vi "Set Admin Password.vi"(8 "error in (no error)":errorcluster, 10 "Set New Admin Password":T1, 11 "Master in":refnum<class "Master.lvclass">) -> (0 "error out":errorcluster, 3 "Master out":refnum<class "Master.lvclass">)   [LabVIEW 2014, in "Master.lvclass"]
uses:
  Master/Master.lvclass
  Master/Master.lvclass/Master.ctl
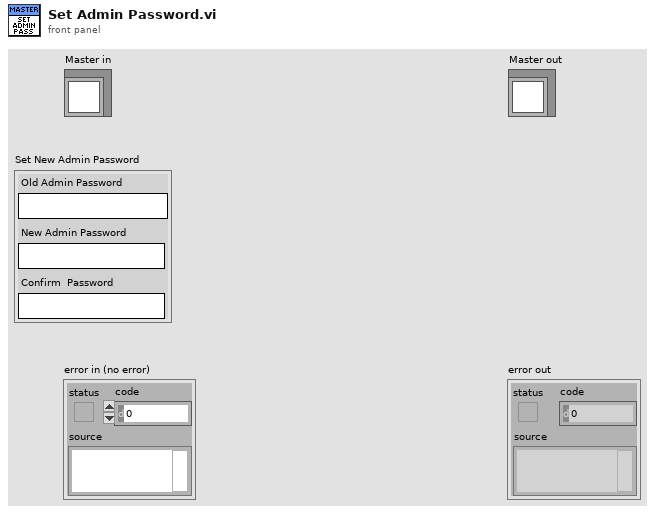
[diagram p1: front panel]
types:
  T1 = cluster{"Old Admin Password":string, "New Admin Password":string, "Confirm  Password":string}
  T2 = cluster{"Admin Password":string, "AutoLogoff":dbl}
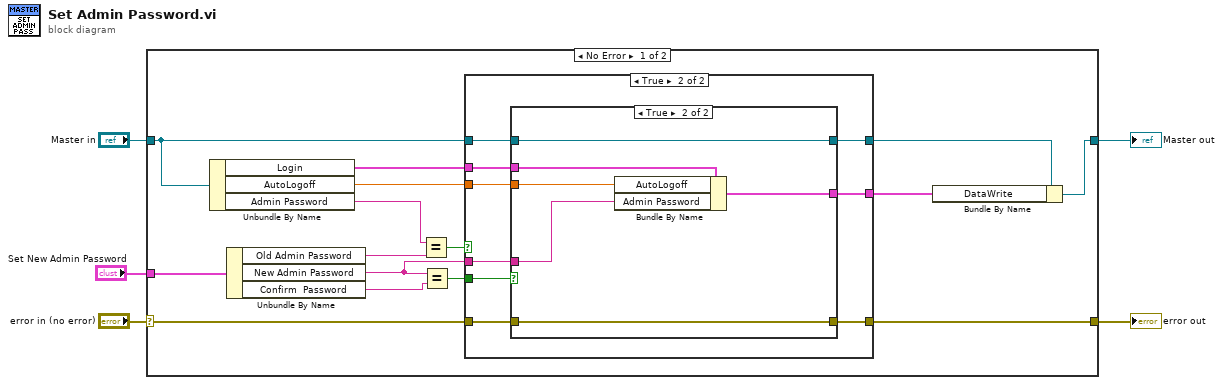
[diagram p0: block diagram]
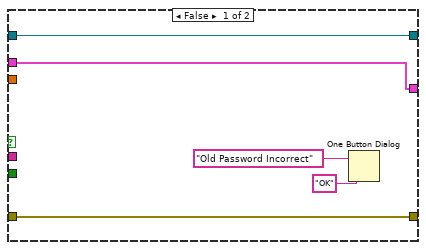
[diagram p2: hidden frame]
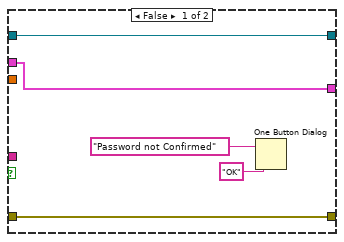
[diagram p3: hidden frame]
diagram:
  n1 = case shown="No Error" "error in (no error)" {
    selector: "error in (no error)" -> [w20 w47]
    tunnel: [w19 w47] -> w4
    tunnel: [w10 w46] -> w2
    tunnel: "Master in" -> [w17 w46]
    tunnel: "Set New Admin Password" -> [w18 _]
    frame No Error {
      n2 = Unbundle By Name(w17) -> ("Login"=w9:T2, "AutoLogoff"=w6:dbl, "Admin Password"=w7:string)
      n3 = Unbundle By Name(w18) -> ("Old Admin Password"=w16:string, "New Admin Password"=w12:string, "Confirm  Password"=w14:string)
      n4 = Equal?(x=w7, y=w16) -> (x = y?=w15:bool)
      n5 = Equal?(x=w12, y=w14) -> (x = y?=w13:bool)
      n6 = case shown="True" w15 {
        tunnel: w20 -> [w25 w34]
        tunnel: [w25 w33] -> w19
        tunnel: w17 -> [w24 w32]
        tunnel: [w24 w31] -> w11
        tunnel: w13 -> [_ w30]
        tunnel: w12 -> [_ w29]
        tunnel: w9 -> [w21 w28]
        tunnel: [w21 w27] -> w8
        tunnel: w6 -> [_ w26]
        frame False {
          n7 = One Button Dialog(message="Old Password Incorrect", button name ("OK")="OK") -> ()  [unwired: 1 out]
        }
        frame True {
          n8 = case shown="True" w30 {
            tunnel: w34 -> [w38 w45]
            tunnel: [w38 w45] -> w33
            tunnel: w32 -> [w39 w41]
            tunnel: [w39 w41] -> w31
            tunnel: w29 -> [_ w42]
            tunnel: w28 -> [w35 w44]
            tunnel: [w35 w43] -> w27
            tunnel: w26 -> [_ w40]
            frame False {
              n9 = One Button Dialog(message="Password not Confirmed", button name ("OK")="OK") -> ()  [unwired: 1 out]
            }
            frame True {
              n10 = Bundle By Name(cluster=w44, "AutoLogoff"=w40, "Admin Password"=w42) -> (w43:T2)
            }
          }
        }
      }
      n11 = Bundle By Name(cluster=w11, "DataWrite"=w8) -> (w10:refnum<class "Master.lvclass">)
    }
    frame Error {
    }
  }
  "error out" <- w4
  "Master out" <- w2
